vi "UIrev2.vi"() -> ()   [LabVIEW 2015]
panel:
  in  "Sensei":bool
  in  "Boolean":bool
  in  "Boolean 10":bool
  in  "Boolean 9":bool
  in  "Boolean 8":bool
  in  "Boolean 7":bool
  in  "Boolean 6":bool
  in  "Boolean 5":bool
  in  "Boolean 4":bool
  in  "Boolean 3":bool
  out "?":i16
  # "Magellan"
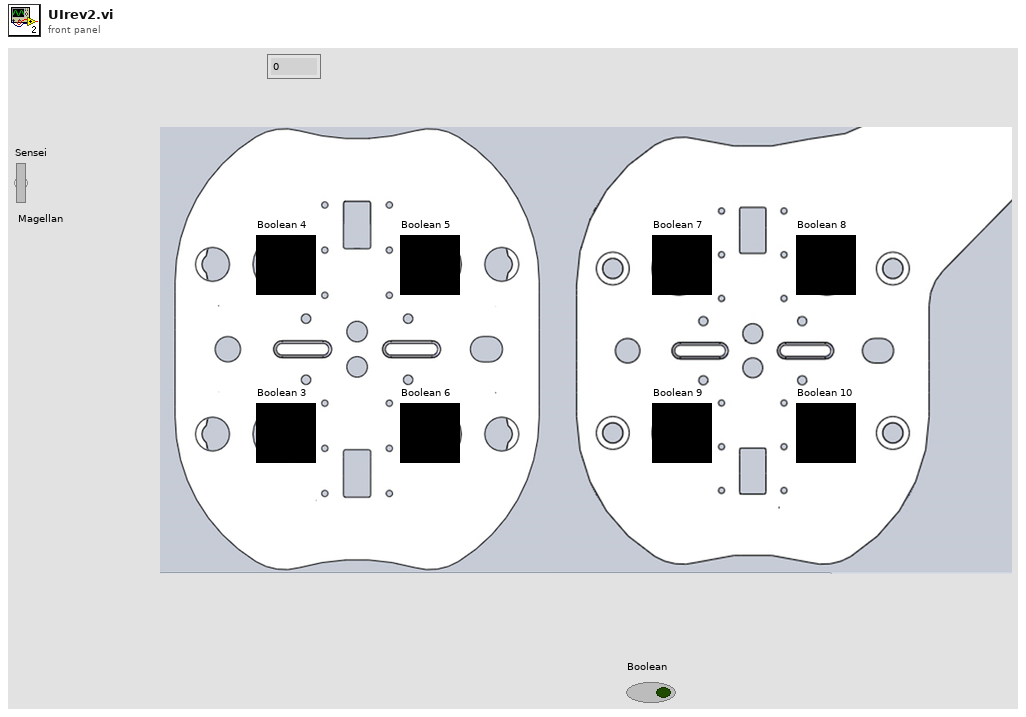
[diagram p1: front panel]
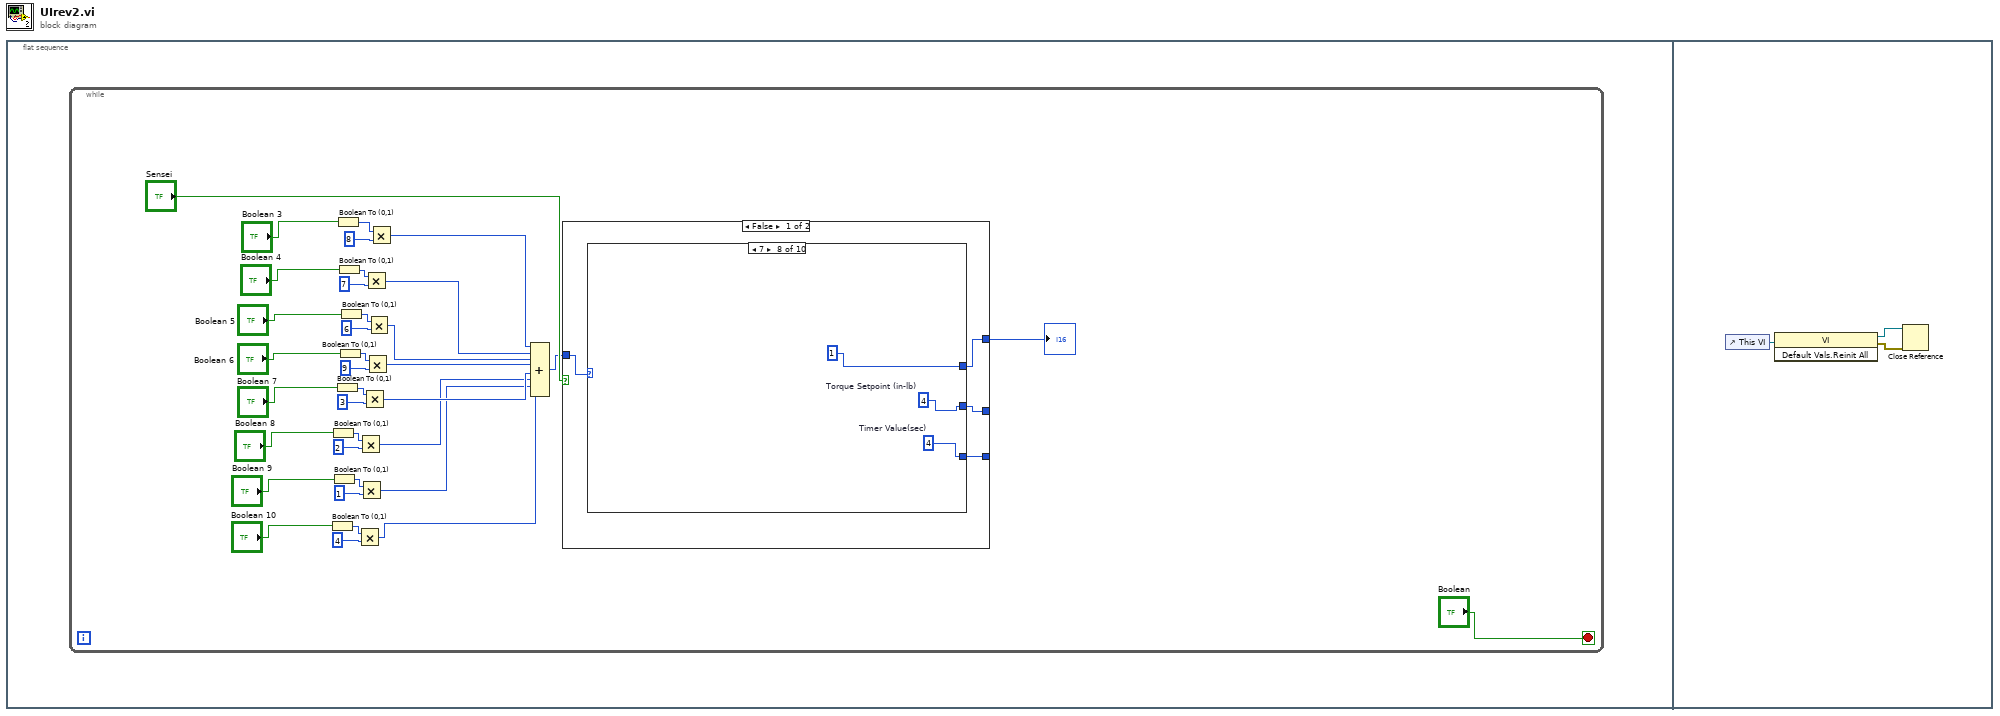
[diagram p0: block diagram]
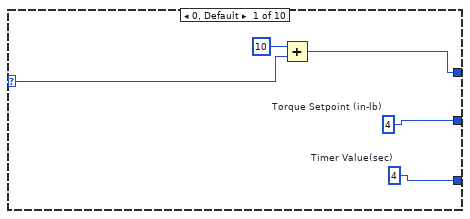
[diagram p2: hidden frame]
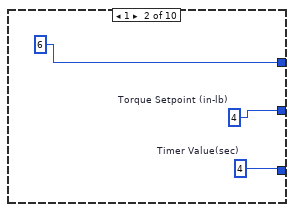
[diagram p3: hidden frame]
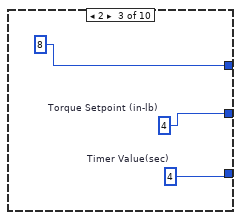
[diagram p4: hidden frame]
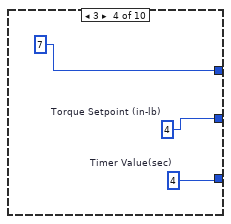
[diagram p5: hidden frame]
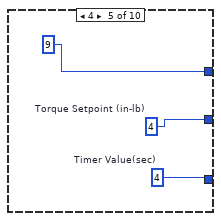
[diagram p6: hidden frame]
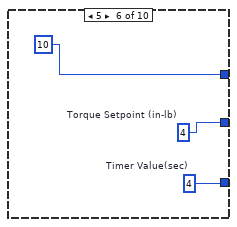
[diagram p7: hidden frame]
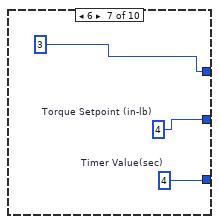
[diagram p8: hidden frame]
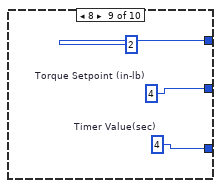
[diagram p9: hidden frame]
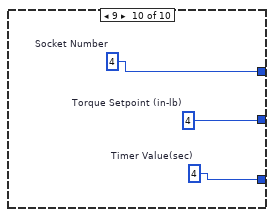
[diagram p10: hidden frame]
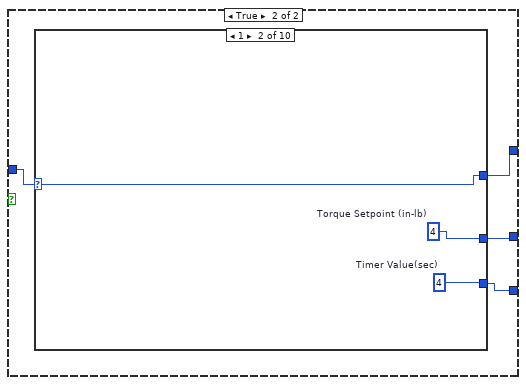
[diagram p11: hidden frame]
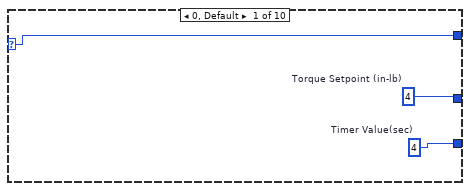
[diagram p12: hidden frame]
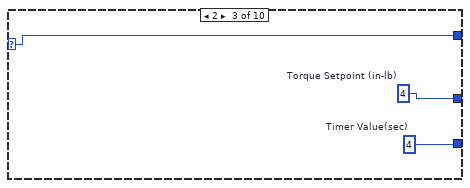
[diagram p13: hidden frame]
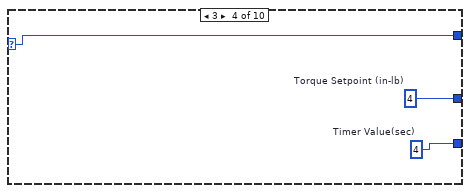
[diagram p14: hidden frame]
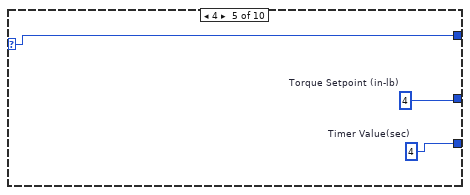
[diagram p15: hidden frame]
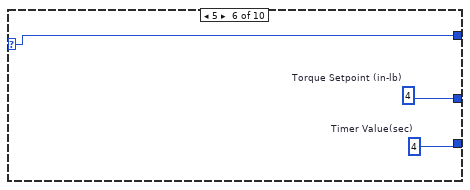
[diagram p16: hidden frame]
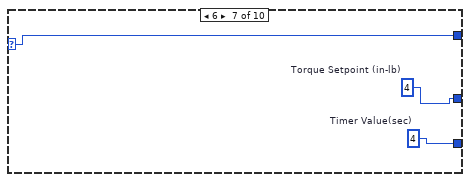
[diagram p17: hidden frame]
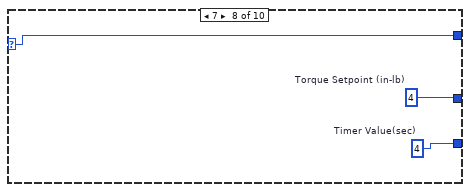
[diagram p18: hidden frame]
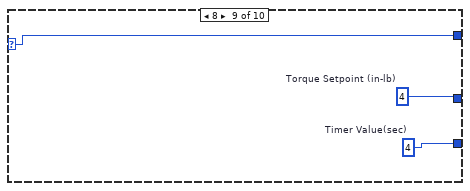
[diagram p19: hidden frame]
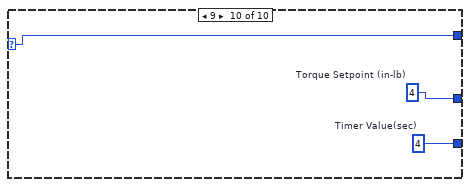
[diagram p20: hidden frame]
diagram:
  n1 = flat-sequence {
    frame #0 {
      n2 = while {
        stop <- "Boolean" stop-if-true
        n3 = Boolean To (0,1)(Boolean="Boolean 10") -> (0, 1=w20:i16)
        n4 = Boolean To (0,1)(Boolean="Boolean 8") -> (0, 1=w24:i16)
        n5 = Boolean To (0,1)(Boolean="Boolean 9") -> (0, 1=w22:i16)
        n6 = Boolean To (0,1)(Boolean="Boolean 7") -> (0, 1=w26:i16)
        n7 = Boolean To (0,1)(Boolean="Boolean 3") -> (0, 1=w36:i16)
        n8 = Boolean To (0,1)(Boolean="Boolean 4") -> (0, 1=w34:i16)
        n9 = Boolean To (0,1)(Boolean="Boolean 6") -> (0, 1=w28:i16)
        n10 = Boolean To (0,1)(Boolean="Boolean 5") -> (0, 1=w30:i16)
        n11 = Multiply(x=w20, y=i16 4) -> (x*y=w5:i16)
        n12 = Multiply(x=w24, y=i16 2) -> (x*y=w7:i16)
        n13 = Multiply(x=w22, y=i16 1) -> (x*y=w6:i16)
        n14 = Multiply(x=w26, y=i16 3) -> (x*y=w8:i16)
        n15 = Multiply(x=w34, y=i16 7) -> (x*y=w11:i16)
        n16 = Multiply(x=w28, y=i16 9) -> (x*y=w9:i16)
        n17 = Multiply(x=w30, y=i16 6) -> (x*y=w10:i16)
        n18 = Multiply(x=w36, y=i16 8) -> (x*y=w12:i16)
        n19 = Compound Arithmetic op=ADD(w12, w11, w10, w9, w8, w7, w6, w5) -> (w1:i16)
        n20 = case shown="False" "Sensei" {
          tunnel: [w40 w76] -> w4
          tunnel: w1 -> [w39 w75]
          tunnel: [w38 w73] -> _
          tunnel: [w37 w74] -> _
          frame False {
            n21 = case shown="7" w39 {
              selector: w39 -> [w43 _ _ _ _ _ _ _ _ _]
              tunnel: [w44 6 ("x") 8 ("x") 7 ("x") 9 ("x") 10 ("x") 3 ("x") 1 ("x") 2 ("x") w72] -> w40
              tunnel: [w42 w47 w50 w53 w56 w59 w62 w65 w68 w71] -> w37
              tunnel: [w41 w46 w49 w52 w55 w58 w61 w64 w67 w70] -> w38
              frame 0, Default {
                w41 = 4  # Timer Value(sec)
                w42 = 4  # Torque Setpoint (in-lb)
                n22 = Add(x=10, y=w43) -> (x+y=w44:i32)
              }
              frame 1 {
                w46 = 4  # Timer Value(sec)
                w47 = 4  # Torque Setpoint (in-lb)
              }
              frame 2 {
                w49 = 4  # Timer Value(sec)
                w50 = 4  # Torque Setpoint (in-lb)
              }
              frame 3 {
                w52 = 4  # Timer Value(sec)
                w53 = 4  # Torque Setpoint (in-lb)
              }
              frame 4 {
                w55 = 4  # Timer Value(sec)
                w56 = 4  # Torque Setpoint (in-lb)
              }
              frame 5 {
                w58 = 4  # Timer Value(sec)
                w59 = 4  # Torque Setpoint (in-lb)
              }
              frame 6 {
                w61 = 4  # Timer Value(sec)
                w62 = 4  # Torque Setpoint (in-lb)
              }
              frame 7 {
                w64 = 4  # Timer Value(sec)
                w65 = 4  # Torque Setpoint (in-lb)
              }
              frame 8 {
                w67 = 4  # Timer Value(sec)
                w68 = 4  # Torque Setpoint (in-lb)
              }
              frame 9 {
                w70 = 4  # Timer Value(sec)
                w71 = 4  # Torque Setpoint (in-lb)
                w72 = 4  # Socket Number
              }
            }
          }
          frame True {
            n23 = case shown="1" w75 {
              selector: w75 -> [w79 w82 w85 w88 w91 w94 w97 w100 w103 w106]
              tunnel: [w79 w82 w85 w88 w91 w94 w97 w100 w103 w106] -> w76
              tunnel: [w78 w81 w84 w87 w90 w93 w96 w99 w102 w105] -> w74
              tunnel: [w77 w80 w83 w86 w89 w92 w95 w98 w101 w104] -> w73
              frame 0, Default {
                w77 = 4  # Timer Value(sec)
                w78 = 4  # Torque Setpoint (in-lb)
              }
              frame 1 {
                w80 = 4  # Timer Value(sec)
                w81 = 4  # Torque Setpoint (in-lb)
              }
              frame 2 {
                w83 = 4  # Timer Value(sec)
                w84 = 4  # Torque Setpoint (in-lb)
              }
              frame 3 {
                w86 = 4  # Timer Value(sec)
                w87 = 4  # Torque Setpoint (in-lb)
              }
              frame 4 {
                w89 = 4  # Timer Value(sec)
                w90 = 4  # Torque Setpoint (in-lb)
              }
              frame 5 {
                w92 = 4  # Timer Value(sec)
                w93 = 4  # Torque Setpoint (in-lb)
              }
              frame 6 {
                w95 = 4  # Timer Value(sec)
                w96 = 4  # Torque Setpoint (in-lb)
              }
              frame 7 {
                w98 = 4  # Timer Value(sec)
                w99 = 4  # Torque Setpoint (in-lb)
              }
              frame 8 {
                w101 = 4  # Timer Value(sec)
                w102 = 4  # Torque Setpoint (in-lb)
              }
              frame 9 {
                w104 = 4  # Timer Value(sec)
                w105 = 4  # Torque Setpoint (in-lb)
              }
            }
          }
        }
        "?" <- w4
      }
    }
    frame #1 {
      n24 = control-ref of="This VI"() -> (w109:refnum<vi>)
      n25 = invoke class="VI" method="Default Vals.Reinit All"(reference=w109) -> (reference out=w108:refnum<vi>, error out=w107:errorcluster)  [unwired: 2 in, 1 out]
      n26 = Close Reference(reference=w108, error in (no error)=w107) -> ()  [unwired: 1 out]
    }
  }
